vi "SwerveAngleMath.vi"(7 "turnSign":dbl, 9 "whRatio":dbl, 10 "Lateral_y":dbl, 11 "Lateral_x":dbl) -> (0 "RRAngle":dbl, 1 "RLAngle":dbl, 2 "FRAngle":dbl, 3 "FLAngle":dbl)   [LabVIEW 2018]
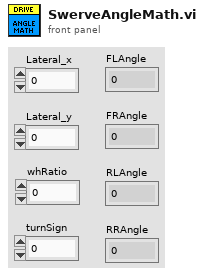
[diagram p1: front panel]
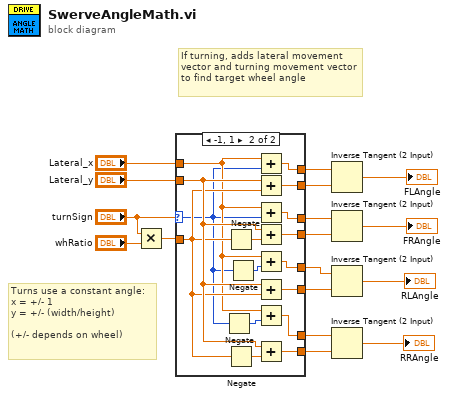
[diagram p0: block diagram]
diagram:
  # "Turns use a constant angle:\nx = +/- 1\ny = +/- (width/height)\n\n(+/- depends on wheel)"
  # "If turning, adds lateral movement vector and turning movement vector to find target wheel angle"
  n1 = Multiply(x="turnSign", y="whRatio") -> (x*y=w3:dbl)
  n2 = case shown="-1, 1" "turnSign" {
    selector: "turnSign" -> [_ w20]
    tunnel: "Lateral_y" -> [w18 w35]
    tunnel: w3 -> [_ w32]
    tunnel: "Lateral_x" -> [w19 w23]
    tunnel: [w19 w31] -> w15
    tunnel: [w18 w30] -> w14
    tunnel: [w19 w29] -> w13
    tunnel: [w18 w28] -> w12
    tunnel: [w19 w27] -> w11
    tunnel: [w18 w26] -> w10
    tunnel: [w19 w25] -> w9
    tunnel: [w18 w24] -> w8
    frame 0, Default {
    }
    frame -1, 1 {
      n3 = Negate(x=w20) -> (-x=w22:i32)
      n4 = Negate(x=w32) -> (-x=w34:dbl)
      n5 = Negate(x=w32) -> (-x=w33:dbl)
      n6 = Negate(x=w20) -> (-x=w21:i32)
      n7 = Add(x=w23, y=w20) -> (x+y=w31:dbl)
      n8 = Add(x=w35, y=w32) -> (x+y=w30:dbl)
      n9 = Add(x=w23, y=w20) -> (x+y=w29:dbl)
      n10 = Add(x=w35, y=w34) -> (x+y=w28:dbl)
      n11 = Add(x=w23, y=w21) -> (x+y=w27:dbl)
      n12 = Add(x=w35, y=w32) -> (x+y=w26:dbl)
      n13 = Add(x=w23, y=w22) -> (x+y=w25:dbl)
      n14 = Add(x=w35, y=w33) -> (x+y=w24:dbl)
    }
  }
  n15 = Inverse Tangent (2 Input)(1:w14, 2:w15) -> (0:→"FLAngle":dbl)
  n16 = Inverse Tangent (2 Input)(1:w12, 2:w13) -> (0:→"FRAngle":dbl)
  n17 = Inverse Tangent (2 Input)(1:w10, 2:w11) -> (0:→"RLAngle":dbl)
  n18 = Inverse Tangent (2 Input)(1:w8, 2:w9) -> (0:→"RRAngle":dbl)
